vi "BuildWaveform_Digital.vi"(10 "DigitalData":bool[](array[boolean]), 11 "SampleRate":dbl) -> (3 "DigitalWaveformOut":digitalwaveform(waveform))   [LabVIEW 2018]
uses:
  <vilib>/Waveform/DWDTOps.llb/DWDT Boolean Array to Digital.vi
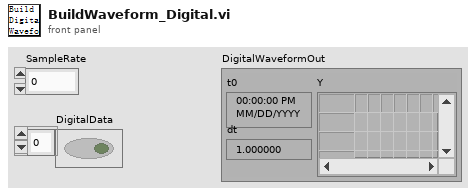
[diagram p1: front panel]
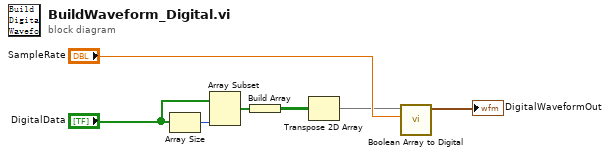
[diagram p0: block diagram]
diagram:
  n1 = Array Size(array="DigitalData") -> (size(s)=w3:i32)
  n2 = Array Subset(array="DigitalData", length=w3) -> (w4:bool[])  [unwired: 1 in]
  n3 = Build Array(w4) -> (w2:bool[][])
  n4 = Transpose 2D Array(2D array=w2) -> (transposed array=w1:bool[][])
  n5 = call-poly <vilib>:"Boolean Array to Digital.vi"("sample rate"="SampleRate", "boolean array"=w1) -> ("digital waveform"=→"DigitalWaveformOut":digitalwaveform)  [unwired: 8 in, 1 out]
